vi "Range_AVS.vi"(10 "old range":i8(ring) items=["no range", "2 Ohms", "20 Ohms", "200 Ohms", "2 kOhms", "20 kOhms", "200 kOhms", "2 MOhms"], 11 "Widerstand":dbl format="%.2f") -> (3 "new range":i8(ring) items=["no range", "2 Ohms", "20 Ohms", "200 Ohms", "2 kOhms", "20 kOhms", "200 kOhms", "2 MOhms"])   [LabVIEW 2016]
panel:
  out "Range value":dbl
  out "Anteil":dbl
  out "iter.Nr":i32
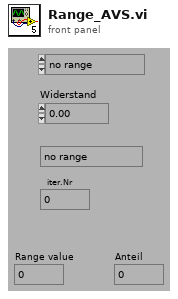
[diagram p1: front panel]
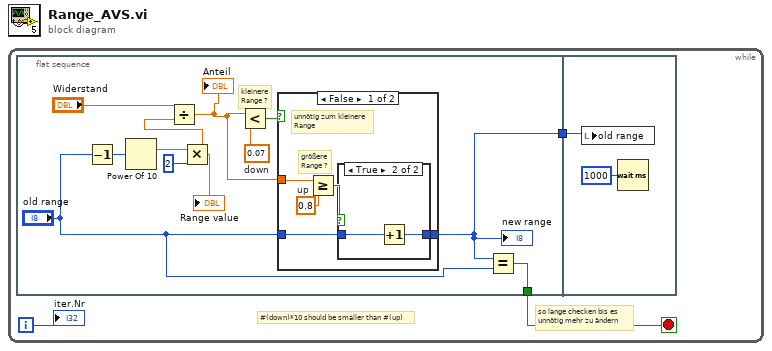
[diagram p0: block diagram]
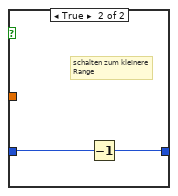
[diagram p3: hidden frame]
diagram:
  n1 = while {
    i -> [w1]
    stop <- w2 stop-if-true
    # "so lange checken bis es \nunnötig mehr zu ändern"
    # "#(down)*10 should be smaller than #(up)"
    n2 = flat-sequence {
      tunnel: [w6] -> w3
      tunnel: [w4] -> w2
      tunnel: w3 -> [w26]
      frame #0 {
        w11 = 0.07  # down
        # "kleinere\nRange ?"
        n3 = Decrement(x="old range") -> (x-1=w7:i8)
        n4 = Power Of 10 ("Potenz von 10")(x=w7) -> (10^x=w14:dbl)
        n5 = Multiply(x=w14, y=2) -> (x*y=w8:dbl)
        "Range value" <- w8
        n6 = Divide(x="Widerstand", y=w8) -> (x/y=w9:dbl)
        "Anteil" <- w9
        n7 = Less?(x=w9, y=w11) -> (x < y?=w10:bool)
        n8 = case shown="False" w10 {
          tunnel: w9 -> [w19 _]
          tunnel: [w15 w23] -> w6
          tunnel: "old range" -> [w16 w24]
          frame False {
            w18 = 0.8  # up
            # "größere\nRange ?"
            # "unnötig zum kleinere\nRange"
            n9 = Greater Or Equal?(x=w19, y=w18) -> (x >= y?=w17:bool)
            n10 = case shown="True" w17 {
              tunnel: w16 -> [w20 w22]
              tunnel: [w20 w21] -> w15
              frame False {
              }
              frame True {
                n11 = Increment(x=w22) -> (x+1=w21:i8)
              }
            }
          }
          frame True {
            # "schalten zum kleinere\nRange"
            n12 = Decrement(x=w24) -> (x-1=w23:i8)
          }
        }
        "new range" <- w6
        n13 = Equal?(x=w6, y="old range") -> (x = y?=w4:bool)
      }
      frame #1 {
        n14 = local write "old range"(w26) -> ()
        n15 = Wait (ms)(milliseconds to wait=1000) -> ()  [unwired: 1 out]
      }
    }
    "iter.Nr" <- w1
  }
